vi "XML429_Database_CloseRefnumArray.vi"(0 "XMLRefnums":refnum<k20>[](array[refnum]), 11 "Error in":errorcluster) -> (15 "Error out":errorcluster)   [LabVIEW 2015, in "AIT 429 System Explorer.lvlib"]
doc: "XML429_Database_CloseRefnumArray"
uses:
  <vilib>/xml/Close Reference(Node).vi
  AIT 429 System Explorer.lvlib
  <vilib>/xml/NI_XML.lvlib
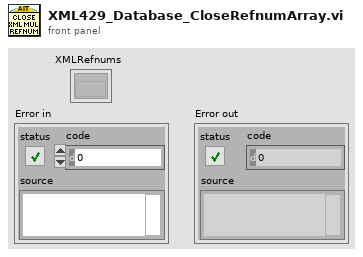
[diagram p1: front panel]
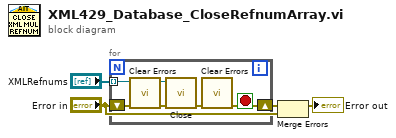
[diagram p0: block diagram]
diagram:
  n1 = for {
    shift-right: [w5] -> w2
    shift-left: "Error in" -> [w8]
    tunnel: "XMLRefnums" -> [w9] mode=indexing
    stop <- w5 stop-if-true
    n2 = call <vilib>:"Clear Errors.vi"("error in (no error)"=w8) -> ("error out"=w7:errorcluster)  [unwired: 5 in, 1 out]
    n3 = call-poly <vilib>:"Close.vi"("error in (no error)"=w7, "node"=w9) -> ("error out"=w6:errorcluster)  [unwired: 7 in]
    n4 = call <vilib>:"Clear Errors.vi"("error in (no error)"=w6) -> ("error out"=w5:errorcluster)  [unwired: 5 in, 1 out]
  }
  n5 = Merge Errors(w2, "Error in") -> (→"Error out":errorcluster)
